vi "Configure Dialog.vi"(8 "error in (no error)":errorcluster, 11 "Configure Trigger Msg.lvclass":refnum<class "Configure Trigger Msg.lvclass">) -> (0 "error out":errorcluster, 2 "Ok?":bool, 3 "Configure Trigger Msg.lvclass":refnum<class "Configure Trigger Msg.lvclass">)   [LabVIEW 2014, in "CS++Scope.lvlib" / "Configure Trigger Msg.lvclass"]
uses:
  Configure Trigger Msg.lvclass
  Configure Trigger Msg.lvclass/Configure Trigger Msg.ctl
panel:
  in  "trigger type (Edge)":i32(ring)=1 items=["Edge"=1, "TV"=5, "Runt"=3, "Glitch"=4, "Width"=2, "AC Line"=7, "Immediate"=6]
  in  "trigger holdoff (500.0 E-9 s)":dbl[unit]
  in  "Cancel Button":bool
  in  "OK Button":bool
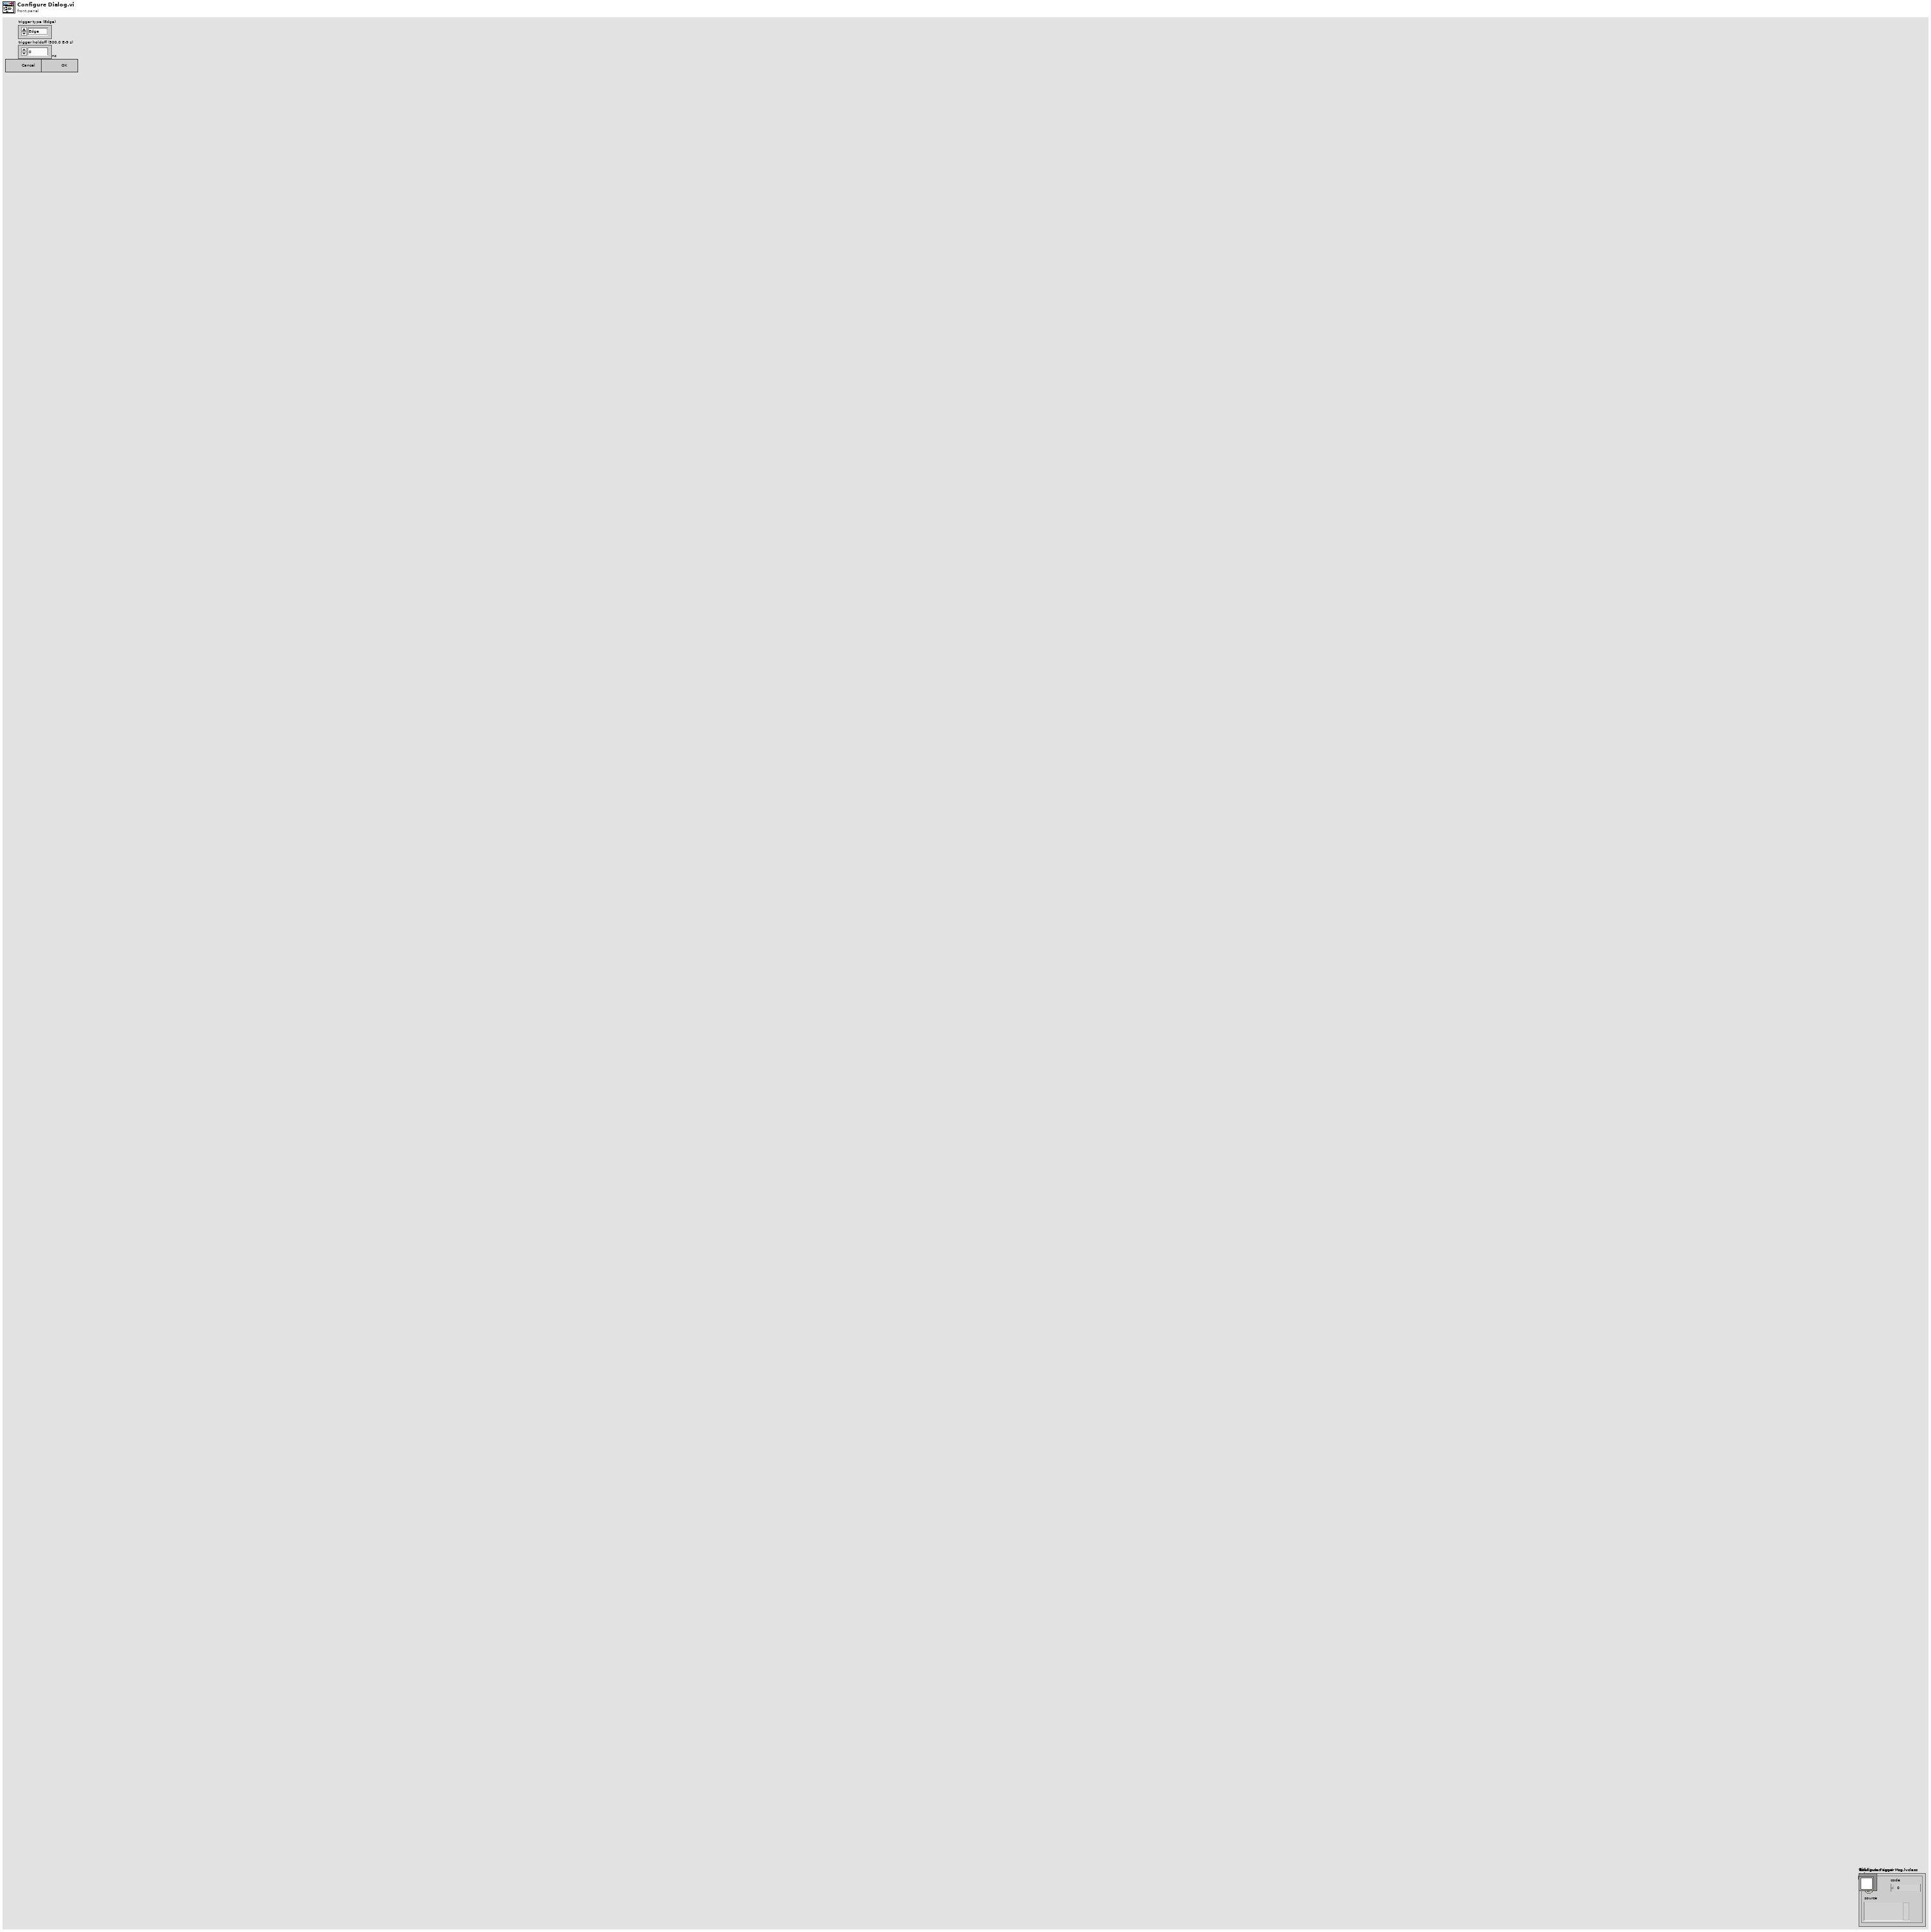
[diagram p1: front panel]
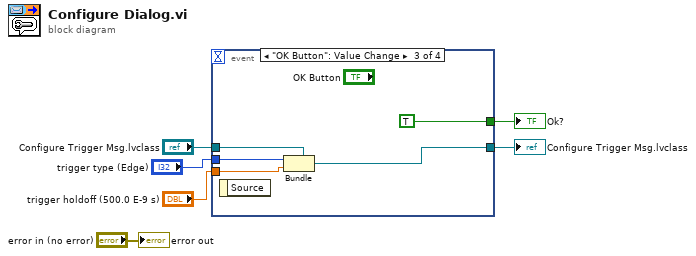
[diagram p0: block diagram]
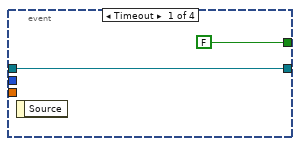
[diagram p2: hidden frame]
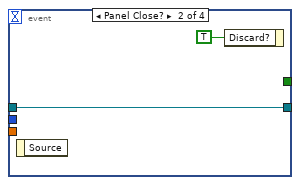
[diagram p3: hidden frame]
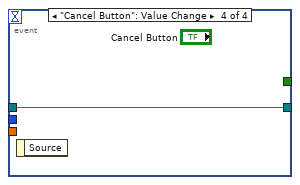
[diagram p4: hidden frame]
diagram:
  n1 = event shown="[2] \"OK Button\": Value Change" {
    selector: _ -> [_ _ _ _]
    dyn-events: _ -> [_ _ _ _]
    timeout: _ -> [_ _ _ _]
    tunnel: [w7 w9 w13 w16] -> w4
    tunnel: "Configure Trigger Msg.lvclass" -> [w7 w9 w15 w16]
    tunnel: [FALSE _ TRUE _] -> w5
    tunnel: "trigger type (Edge)" -> [_ _ w12 _]
    tunnel: "trigger holdoff (500.0 E-9 s)" -> [_ _ w11 _]
    event Timeout {
      n2 = event-data() -> ()  [unwired: 1 in, 1 out]
    }
    event Panel Close? {
      n3 = event-data() -> ()  [unwired: 1 in, 1 out]
      n4 = event-data ("Event Filter Node")("Discard?"=TRUE) -> ()  [unwired: 1 in, 1 out]
    }
    event "OK Button": Value Change {
      n5 = event-data() -> ()  [unwired: 1 in, 1 out]
      n6 = Bundle ("Main-Bundler")(cluster=w15, w12, w11) -> (w13:refnum<class "Configure Trigger Msg.lvclass">)
    }
    event "Cancel Button": Value Change {
      n7 = event-data() -> ()  [unwired: 1 in, 1 out]
    }
  }
  "Ok?" <- w5
  "Configure Trigger Msg.lvclass" <- w4
  "error out" <- "error in (no error)"
